vi "Write STATUS cluster.vi"(8 "error in (no error)":errorcluster, 10 "STATUS cluster":T1={"OBSERVER"="", "OBJECT"="", "CTRLINTE"="S4GUI", "PROJID"="", "SYNCMODE"="SYNC", "INSTMODE"="PHOT", "FILTER"="CLEAR", "OBSTYPE"="", "CHANNEL 1"=FALSE, "CHANNEL 2"=FALSE, "CHANNEL 3"=FALSE, "CHANNEL 4"=FALSE, "TCSMODE"=FALSE, "COMMENT"="", "BROKER"="S4GUI"}, 11 "Publisher in":refnum<class "Publisher.lvclass">) -> (0 "error out":errorcluster, 3 "Publisher out":refnum<class "Publisher.lvclass">)   [LabVIEW 2018, in "Publisher.lvclass"]
uses:
  Publisher.lvclass
  Publisher.lvclass/Publisher.ctl
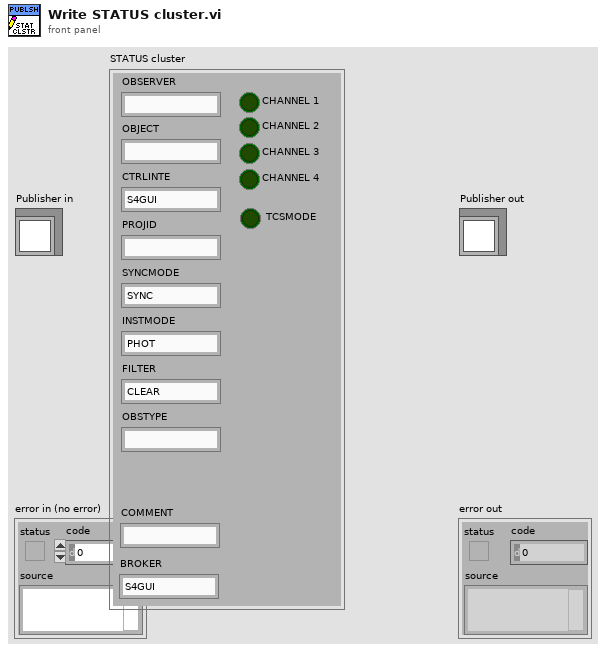
[diagram p1: front panel]
types:
  T1 = cluster{"OBSERVER":string, "OBJECT":string, "CTRLINTE":string, "PROJID":string, "SYNCMODE":string, "INSTMODE":string, "FILTER":string, "OBSTYPE":string, "CHANNEL 1":bool, "CHANNEL 2":bool, "CHANNEL 3":bool, "CHANNEL 4":bool, "TCSMODE":bool, "COMMENT":string, "BROKER":string}
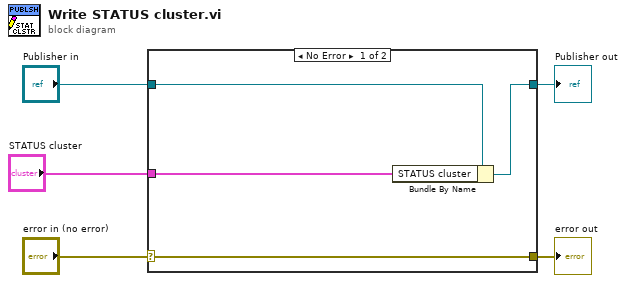
[diagram p0: block diagram]
diagram:
  n1 = case shown="No Error" "error in (no error)" {
    selector: "error in (no error)" -> [w9 w10]
    tunnel: [w9 w10] -> w4
    tunnel: [w7 w11] -> w2
    tunnel: "Publisher in" -> [w8 w11]
    tunnel: "STATUS cluster" -> [w6 _]
    frame No Error {
      n2 = Bundle By Name(cluster=w8, "STATUS cluster"=w6) -> (w7:refnum<class "Publisher.lvclass">)
    }
    frame Error {
    }
  }
  "error out" <- w4
  "Publisher out" <- w2
